vi "AIT 1553 - Build BC Message Properties.vi"(8 "error in (no error)":errorcluster, 10 "BC_Message":T1) -> (0 "error out":errorcluster, 1 "Tx-Rx  (T=Tx)":bool, 2 "name":string, 4 "Prop Names":string[](array[string]), 6 "Prop Values":variant[](array[variant]))   [LabVIEW 2011, in "AIT 1553 Custom Device.lvlib"]
uses:
  AIT 1553 Custom Device.lvlib
  Controls/1553_BC_Message.ctl
  Controls/1553 Param.ctl
  Controls and Global/Global.vi
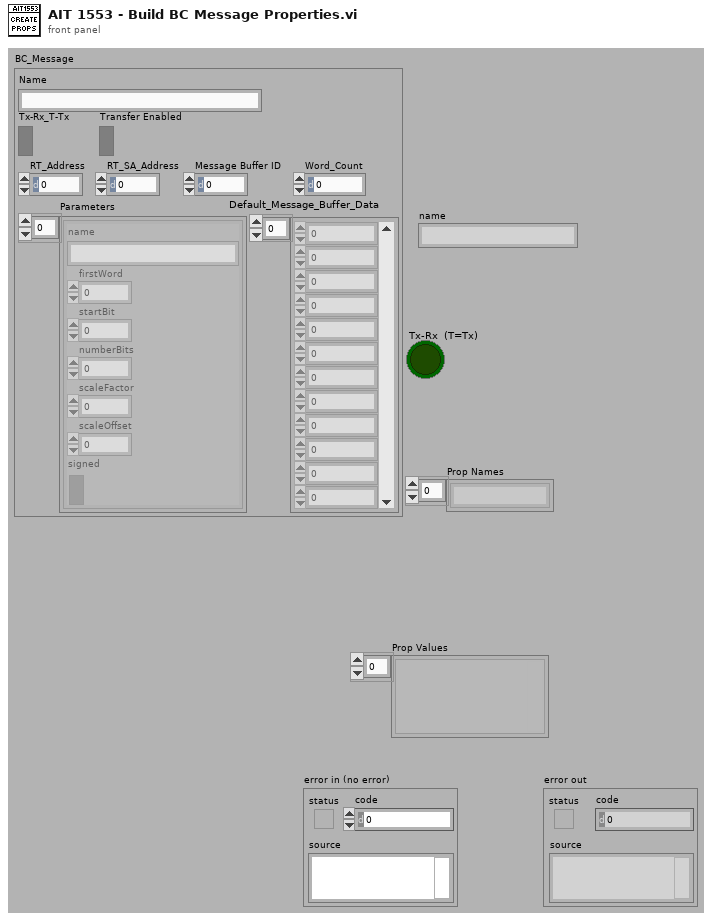
[diagram p1: front panel]
types:
  T1 = typedef "AIT 1553 Custom Device.lvlib/1553_BC_Message.ctl" = cluster{"Name":string, "Tx-Rx_T-Tx":bool, "RT_Address":u8, "RT_SA_Address":u8, "Parameters":T2[], "Transfer Enabled":bool, "Message Buffer ID":u16, "Default_Message_Buffer_Data":u16[], "Word_Count":u8}
  T2 = typedef "AIT 1553 Custom Device.lvlib/1553 Param.ctl" = cluster{"name":string, "firstWord":i32, "startBit":i32, "numberBits":i32, "scaleFactor":dbl, "scaleOffset":dbl, "signed":bool}
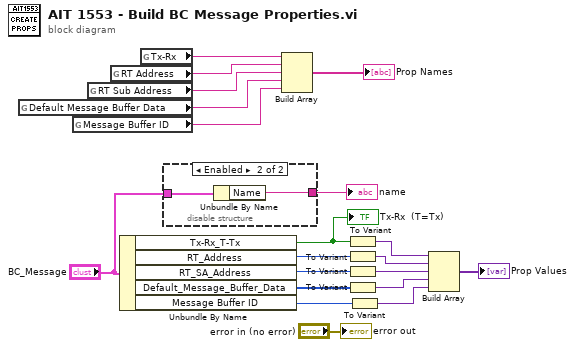
[diagram p0: block diagram]
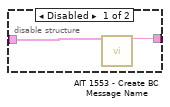
[diagram p2: hidden frame]
diagram:
  n1 = global read "Global.vi" "Default Message Buffer Data"() -> (w9:string)
  n2 = global read "Global.vi" "Message Buffer ID"() -> (w6:string)
  n3 = global read "Global.vi" "RT Sub Address"() -> (w18:string)
  n4 = global read "Global.vi" "RT Address"() -> (w5:string)
  n5 = Unbundle By Name("BC_Message") -> ("Tx-Rx_T-Tx"=w12:bool, "RT_Address"=w13:u8, "RT_SA_Address"=w14:u8, "Default_Message_Buffer_Data"=w8:u16[], "Message Buffer ID"=w4:u16)
  "Tx-Rx  (T=Tx)" <- w12
  n6 = global read "Global.vi" "Tx-Rx"() -> (w20:string)
  n7 = disable-structure shown="Enabled" {
    disable-tunnel: "BC_Message" -> [w22 w24]
    disable-tunnel: [w21 w23] -> w1
    frame Disabled {
      n8 = call "AIT 1553 - Create BC Message Name.vi"("BC_Message"=w22) -> ("Message Name"=w21:string)  [unwired: 13 in, 1 out]
    }
    frame Enabled {
      n9 = Unbundle By Name(w24) -> ("Name"=w23:string)
    }
  }
  "name" <- w1
  n10 = Build Array(w20, w5, w18, w9, w6) -> (→"Prop Names":string[])
  n11 = To Variant(anything=w12) -> (Variant=w15:variant)
  n12 = To Variant(anything=w13) -> (Variant=w16:variant)
  n13 = To Variant(anything=w14) -> (Variant=w17:variant)
  n14 = To Variant(anything=w8) -> (Variant=w7:variant)
  n15 = To Variant(anything=w4) -> (Variant=w3:variant)
  n16 = Build Array(w15, w16, w17, w7, w3) -> (→"Prop Values":variant[])
  "error out" <- "error in (no error)"
